vi "Command.vi"(8 "error in (no error)":errorcluster, 9 "command value (no value)":string, 10 "command":string, 11 "MKS MF1 in":refnum<class "PL MKS MF1 USB.lvclass">) -> (0 "error out":errorcluster, 1 "response value":string, 2 "valve mode":u8(ring) items=["normal", "closed", "purge"], 3 "MKS MF1 out":refnum<class "PL MKS MF1 USB.lvclass">)   [LabVIEW 2015, in "PL MKS MF1 USB.lvclass"]
doc: "Sends <b>command</b> with <b>command value</b> to device and returns <b>valve mode</b> and <b>response value</b>."
uses:
  PL MKS MF1 USB.lvclass
  PL MKS MF1 USB.lvclass/PL MKS MF1 USB.ctl
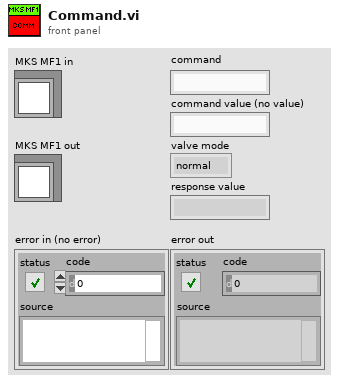
[diagram p1: front panel]
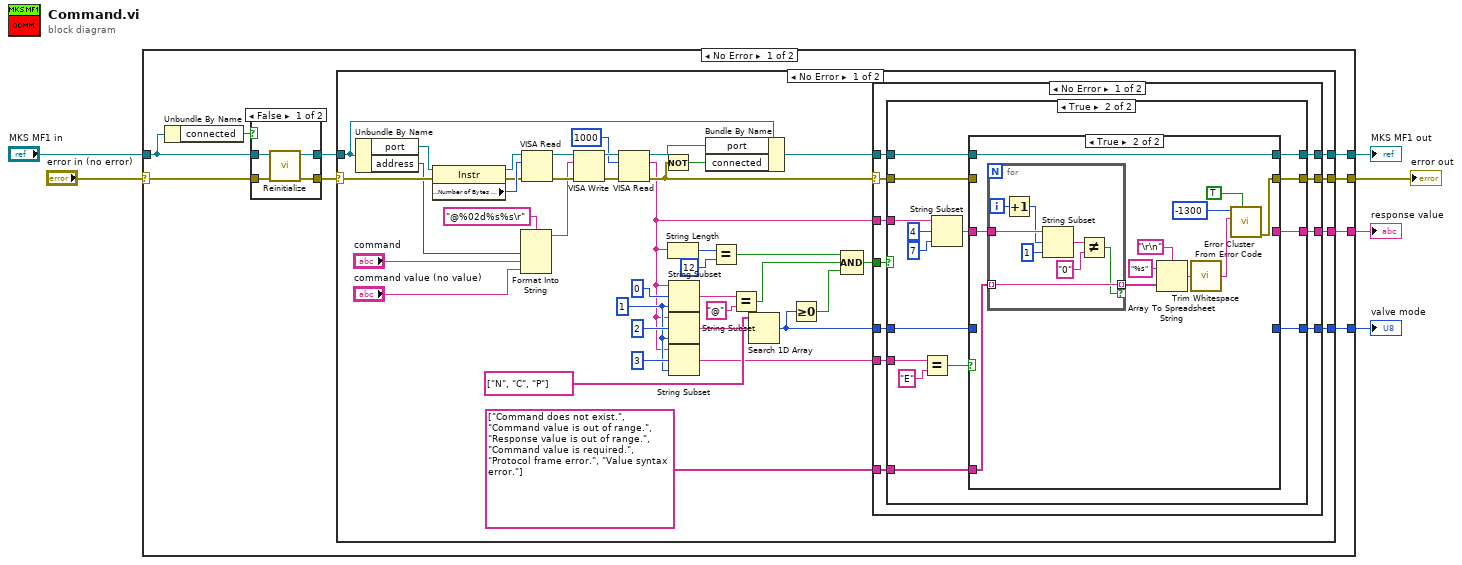
[diagram p0: block diagram]
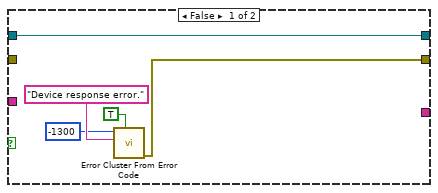
[diagram p2: hidden frame]
diagram:
  n1 = case shown="No Error" "error in (no error)" {
    selector: "error in (no error)" -> [w13 w123]
    tunnel: "MKS MF1 in" -> [w14 w122]
    tunnel: [w10 w123] -> w3
    tunnel: [w9 w122] -> w4
    tunnel: [w8 _] -> w2
    tunnel: [w7 _] -> w1
    frame No Error {
      n2 = Unbundle By Name(w14) -> ("connected"=w15:bool)
      n3 = case shown="False" w15 {
        tunnel: w14 -> [w119 w121]
        tunnel: w13 -> [w118 w120]
        tunnel: [w117 w121] -> w11
        tunnel: [w116 w120] -> w12
        frame False {
          n4 = call "Reinitialize.vi"("error in (no error)"=w118, "MKS MF1 in"=w119) -> ("error out"=w116:errorcluster, "MKS MF1 out"=w117:refnum<class "PL MKS MF1 USB.lvclass">)  [unwired: 8 in]
        }
        frame True {
        }
      }
      n5 = case shown="No Error" w12 {
        selector: w12 -> [w46 w115]
        tunnel: w11 -> [w54 w114]
        tunnel: [w25 w115] -> w10
        tunnel: [w20 w114] -> w9
        tunnel: [w23 _] -> w8
        tunnel: [w22 _] -> w7
        frame No Error {
          w34 = 1 ("length (rest)")
          n6 = Unbundle By Name(w54) -> ("port"=w47:refnum<visa-resource-name>, "address"=w43:u8)
          n7 = property class="Instr"(reference=w47, error in=w46) -> (reference out=w50:refnum<visa-resource-name>, error out=w45:errorcluster, "Serial Settings:Number of Bytes at Serial Port"=w51:u32)
          n8 = Format Into String(format string="@%02d%s%s\r", w43, "command", "command value (no value)") -> (resulting string=w41:string)  [unwired: 2 in, 1 out]
          n9 = VISA Read(VISA resource name=w50, byte count=w51, error in (no error)=w45) -> (VISA resource name out=w49:refnum<visa-resource-name>, error out=w48:errorcluster)  [unwired: 2 out]
          n10 = VISA Write(VISA resource name=w49, write buffer=w41, error in (no error)=w48) -> (VISA resource name out=w57:refnum<visa-resource-name>, error out=w56:errorcluster)  [unwired: 1 out]
          n11 = VISA Read(VISA resource name=w57, byte count=u32 1000, error in (no error)=w56) -> (VISA resource name out=w53:refnum<visa-resource-name>, read buffer=w18:string, error out=w27:errorcluster)  [unwired: 1 out]
          n12 = Not(x=w27) -> (.not. x?=w52:bool)
          n13 = String Length(string=w18) -> (length=w40:i32)
          n14 = String Subset(string=w18, offset (0)=0, length (rest)=w34) -> (substring=w33:string)
          n15 = String Subset(string=w18, offset (0)=2, length (rest)=w34) -> (substring=w30:string)
          n16 = String Subset(string=w18, offset (0)=3, length (rest)=w34) -> (substring=w16:string)
          n17 = Bundle By Name(cluster=w54, "port"=w53, "connected"=w52) -> (w21:refnum<class "PL MKS MF1 USB.lvclass">)
          n18 = Equal?(x=w40, y=12) -> (x = y?=w38:bool)
          n19 = Equal?(x=w33, y="@") -> (x = y?=w31:bool)
          n20 = Search 1D Array(1D array=string[] ["N", "C", "P"], element=w30) -> (index of element=w24:i32)  [unwired: 1 in]
          n21 = Greater Or Equal To 0?(x=w24) -> (x >= 0?=w17:bool)
          n22 = Compound Arithmetic op=AND(w38, w31, w17) -> (w26:bool)
          n23 = case shown="No Error" w27 {
            selector: w27 -> [w64 w113]
            tunnel: w26 -> [w68 _]
            tunnel: [w67 w113] -> w25
            tunnel: w24 -> [w66 _]
            tunnel: w18 -> [w65 _]
            tunnel: [w63 _] -> w23
            tunnel: [w62 _] -> w22
            tunnel: w21 -> [w61 w112]
            tunnel: [w60 w112] -> w20
            tunnel: string[] ["Command does not exist.", "Command value is out of range.", "Response value is out of range.", "Command value is required.", "Protocol frame error.", "Value syntax error."] -> [w59 _]
            tunnel: w16 -> [w58 _]
            frame No Error {
              n24 = case shown="True" w68 {
                tunnel: [w70 w88] -> w67
                tunnel: w66 -> [_ w84]
                tunnel: w65 -> [_ w87]
                tunnel: w64 -> [_ w86]
                tunnel: [_ w85] -> w63
                tunnel: [_ w83] -> w62
                tunnel: w61 -> [w69 w82]
                tunnel: [w69 w81] -> w60
                tunnel: w59 -> [_ w80]
                tunnel: w58 -> [_ w74]
                frame False {
                  n25 = call <vilib>:"Error Cluster From Error Code.vi"("show call chain? (False)"=TRUE, "error message (\"\")"="Device response error." ("format string"), "error code (0)"=-1300) -> ("error out"=w70:errorcluster)  [unwired: 6 in]
                }
                frame True {
                  n26 = Equal?(x=w74, y="E") -> (x = y?=w75:bool)
                  n27 = String Subset(string=w87, offset (0)=4, length (rest)=7 ("length (rest)")) -> (substring=w77:string)
                  n28 = case shown="True" w75 {
                    tunnel: [w89 _] -> w85
                    tunnel: w82 -> [w92 w103]
                    tunnel: [w92 w103] -> w81
                    tunnel: w84 -> [w91 _]
                    tunnel: [w91 _] -> w83
                    tunnel: w86 -> [w90 _]
                    tunnel: [w90 w93] -> w88
                    tunnel: w77 -> [w89 w102]
                    tunnel: w80 -> [_ w101]
                    frame False {
                    }
                    frame True {
                      n29 = for {
                        tunnel: w102 -> [w111]
                        tunnel: w101 -> [w105] mode=indexing
                        tunnel: [w105] -> w100 mode=indexing if=w104
                        i -> [w110]
                        n30 = Increment(x=w110) -> (x+1=w109:i32)
                        n31 = String Subset(string=w111, offset (0)=w109, length (rest)=1 ("length (rest)")) -> (substring=w107:string)
                        n32 = Not Equal?(x=w107, y="0") -> (x != y?=w104:bool)
                      }
                      n33 = Array To Spreadsheet String(delimiter (Tab)="\r\n", array=w100, 3:"%s" ("format string")) -> (spreadsheet string=w95:string)
                      n34 = call <vilib>:"Trim Whitespace.vi"("string"=w95) -> ("trimmed string"=w94:string)  [unwired: 1 in]
                      n35 = call <vilib>:"Error Cluster From Error Code.vi"("show call chain? (False)"=TRUE, "error message (\"\")"=w94, "error code (0)"=-1300) -> ("error out"=w93:errorcluster)  [unwired: 6 in]
                    }
                  }
                }
              }
            }
            frame Error {
            }
          }
        }
        frame Error {
        }
      }
    }
    frame Error {
    }
  }
  "MKS MF1 out" <- w4
  "error out" <- w3
  "valve mode" <- w1
  "response value" <- w2
